vi "Airflow_Simulator_Main.vi"() -> ()   [LabVIEW 2025]
uses:
  controls/Tuners.ctl
  controls/Constants.ctl
  controls/Design_Results.ctl
  controls/UI Data.ctl
  Settings/Settings.ctl
  Acquisition/Hardware Configuration.ctl
  Acquisition/Signal Type.ctl
  Logging/Logging Configuration.ctl
  controls/UI State.ctl
  controls/State_Machine_Steps.ctl
  support/Message Queue/Enqueue Message (Single).vi
  support/Message Queue/Enqueue Message (Array).vi
  <vilib>/Utility/error.llb/Error Cluster From Error Code.vi
  <vilib>/ErrorRing/Error Ring.xnode
  Settings/Settings.lvlib
  support/Message Queue/Message Queue.lvlib
  Settings/Settings Dialog.vi
  support/User Event - Stop/User Event - Stop.lvlib
  Acquisition/Acquisition.lvlib
  Logging/Logging.lvlib
panel:
  in  "Tab Control":T1(tab)
  in  "Design Constants":T2={"P_amb (psia)"=14.7, "T_in (Deg F)"=530.0, "R_air (ft*lbf)/(lbm*R)"=53.35, "g_c (lbm*ft)/(lbf*s^2)"=32.17, "specific heat ratio"=1.4, "Viscousity (lbm)/(ft*s)"=1.21e-05, "Cd"=0.61, "Mass Flow (lbm/min) vs. Pressure Drop (inH2O) - Real Data"=[[0.5, 0.0149], [1.0, 0.0619], [1.5, 0.139], [2.0, 0.249], [2.5, 0.385], [3.5, 0.73]]} {"Mass Flow (lbm/min) vs. Pressure Drop (inH2O) - Real Data" format="%_3g"; "P_amb (psia)" format="%#_4g"}
  in  "Submit to DB":bool
  out "Design Results":T3 {"Design Results"."Optimized Inlet \nOrifice Diameter (in)" format="%#_3g"}
  in  "Tuners":T4 {"OAR" items=["0.92"=0.92, "0.93"=0.93, "0.94"=0.94, "0.95"=0.95, "0.96"=0.96]; "D_h (in)" items=["0.0625"=0.0625, "0.125"=0.125, "0.250"=0.25]; "Diameter (in)" min=0.1 max=6.0 scale=0.0..6.0 scale format="%#_3g"; "Length (in)" min=0.1 max=5.0 scale=0.0..6.0 scale format="%#_3g"; "Outlet Diameter (in)" min=0.1 max=5.0 scale=0.0..5.0 scale format="%#_3g"; "Inlet Diameter (in)" min=0.1 max=5.0 scale=0.0..5.0}
  in  "Start":bool
  in  "Settings":bool
  in  "Stop":bool
  in  "Exit":bool
  out "Status":string
  # "AIRFLOW SIMULATOR"
  # "Temperature_Tap"
  # "Pressure_Tap"
  # "Mass_flowrate"
  # "Outlet_Diameter"
  # "Inlet_Diameter"
  # "Pressure_Ambient"
  # "Pressure_Inlet"
  # "Pipe_Diameter"
  # "Temperature_Inlet"
  # "Honeycomb_Length"
  # "Temperature_Ambient"
  # "DESIGN PARAMETERS AND PROPERTIES"
  # "PIPE"
  # "ORIFICES"
  # "HONEYCOMB"
  # "AIR PROPERTIES"
  # "**Outlet_Diameter"
  # "**Pipe_Diameter"
  # "**D_h"
  # "Temperature_Inlet (Deg F) = 70"
  # "**Inlet_Diameter"
  # "**OAR"
  # "R_air (ft*lbf)/(lbm*R) = 53.35"
  # "Cd_orifice  = 0.61"
  # "**Honeycomb_Length"
  # "specific heat ratio = 1.40"
  # "Viscousity (lbm)/(ft*s) = 1.21E-5"
  # "**To Be Determine Using Design Mode"
  # "Pressure_Ambient (psia) = 14.7"
  # "Pressure_Inlet"
  # "Empirical Flow Path Data"
  # "Mass Flow\n (lbm/min)"
  # "Pressure Drop \n    (inH2O)"
  # "Simulator Fit"
  # "Empirical Fit"
  # "="
  # "P"
  # "* X"
  # "P"
  # "="
  # "* X"
  # "drop"
  # "drop"
  # "Honeycomb Parameters"
  # "Orifice Parameters"
  # "Pipe Parameters"
  # "AIRFLOW SIMULATOR"
  # "Mass_flowrate"
  # "Pipe_Diameter"
  # "Outlet_Diameter"
  # "Inlet_Diameter"
  # "Honeycomb_Length"
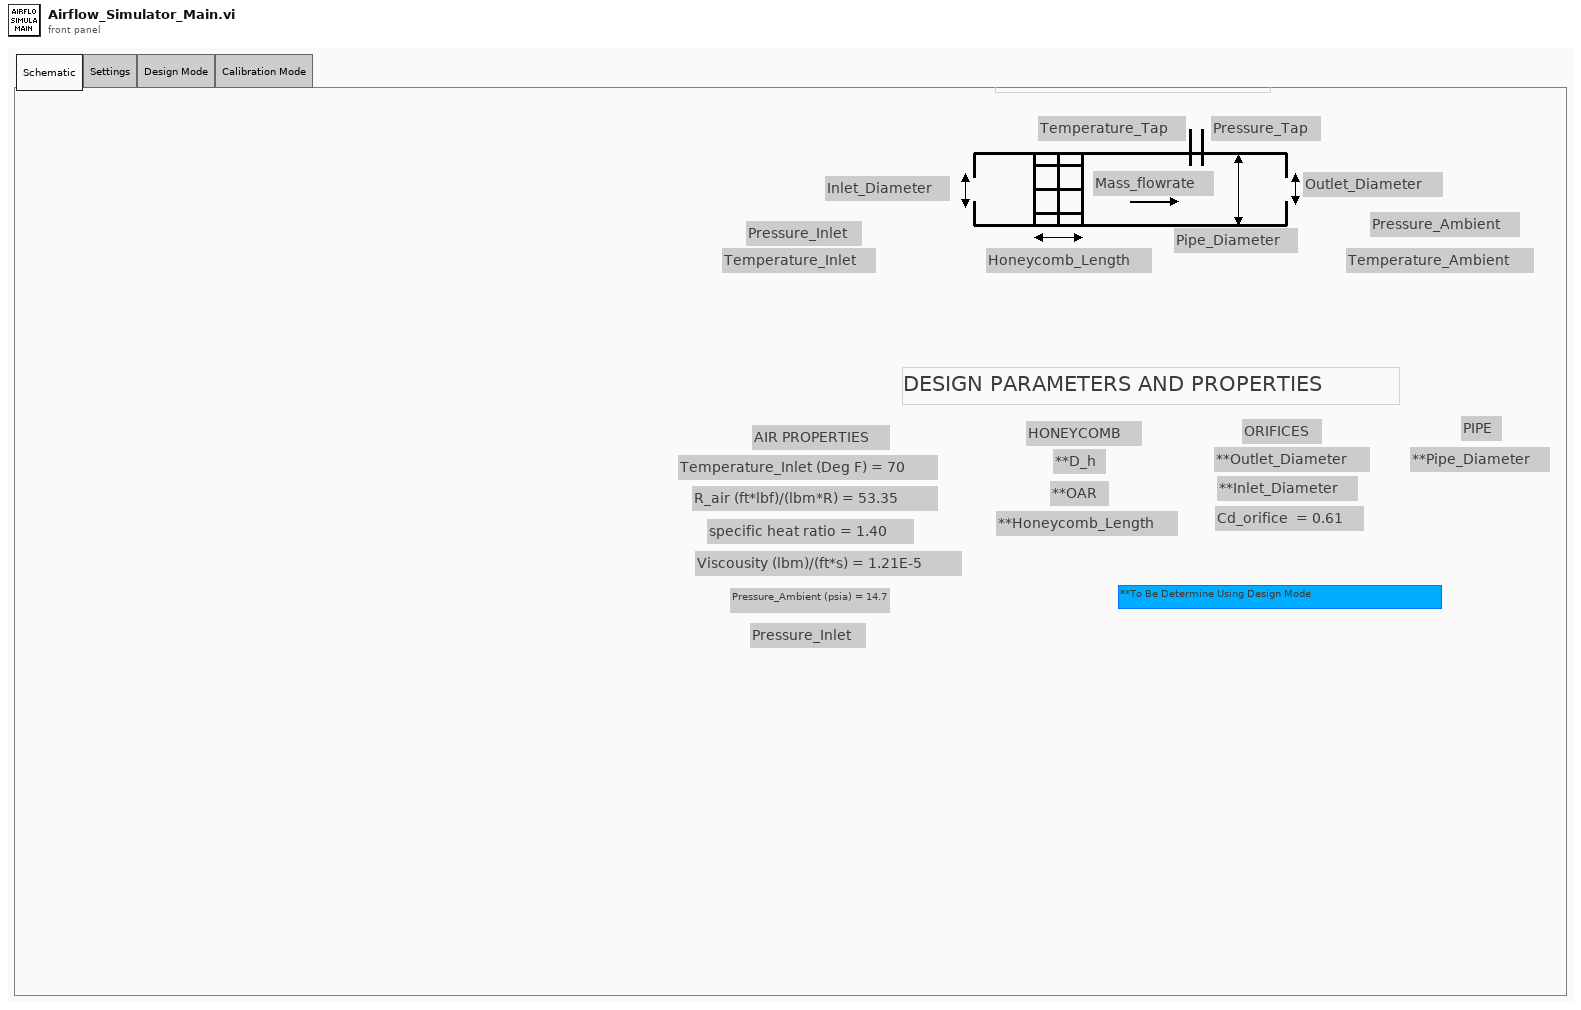
[diagram p1: front panel]
types:
  T1 = enum32{"Schematic", "Settings", "Design Mode", "Calibration Mode"}
  T2 = typedef "Constants.ctl" = cluster{"P_amb (psia)":dbl, "T_in (Deg F)":dbl, "R_air (ft*lbf)/(lbm*R)":dbl, "g_c (lbm*ft)/(lbf*s^2)":dbl, "specific heat ratio":dbl, "Viscousity (lbm)/(ft*s)":dbl, "Cd":dbl, "Mass Flow (lbm/min) vs. Pressure Drop (inH2O) - Real Data":dbl[][]}
  T3 = typedef "Design_Results.ctl" = cluster{"Design Results":cluster{"Model Validation: Simulated vs. Empirical Airflow Data":cluster{dbl[], dbl[]}[], "Amplitude - Empirical":string, "Power - Empirical":string, "Amplitude - Sim":string, "Power - Sim":string, "Flow Type":u32, "Optimized Inlet \nOrifice Diameter (in)":dbl, "Flow Type Name":string}}
  T4 = typedef "Tuners.ctl" = cluster{"Inlet Diameter (in)":dbl, "Outlet Diameter (in)":dbl, " Length (in)":dbl, "   Diameter (in)":dbl, "D_h (in)":dbl, "OAR":dbl, "Run Optimizer":bool}
  T5 = typedef "State_Machine_Steps.ctl" = enum16{"Init", "Event", "Design", "Calibrate", "Stop"}
  T6 = typedef "UI State.ctl" = enum16{"Idle", "Acquiring and Logging", "Waiting for Exit", "Waiting for Exit (Acq Stopped)", "Waiting for Exit (Log Stopped)", "Waiting for Stop", "Waiting for Stop (Acq Stopped)", "Waiting for Stop (Log Stopped)"}
  T7 = typedef "Settings.lvlib/Settings.ctl" = cluster{"Hardware Configuration":T8, "Logging Configuration":T10}
  T8 = typedef "Acquisition.lvlib/Hardware Configuration.ctl" = cluster{"HW Refnum <Replace Me>":string, "Signal Type <Replace Me>":T9}
  T9 = typedef "Acquisition.lvlib/Signal Type.ctl" = enum16{"Sine Wave", "Square with Noise"}
  T10 = typedef "Logging.lvlib/Logging Configuration.ctl" = cluster{"Log File Base Path":path, "TDMS File Reference":refnum<k34>}
  T11 = typedef "UI Data.ctl" = cluster{"Start Ref":refnum<vi>, "Stop Ref":refnum<vi>, "Settings Ref":refnum<vi>, "Exit Ref":refnum<vi>, "Status Ref":refnum<vi>, "Data Ref":refnum<vi>}
  T12 = typedef "Message Queue.lvlib/All Message Queues.ctl" = cluster{"UI":refnum<queue>, "Acquisition":refnum<queue>, "Logging":refnum<queue>, "Design":refnum<queue>, "Display":refnum<queue>, "Database":refnum<queue>}
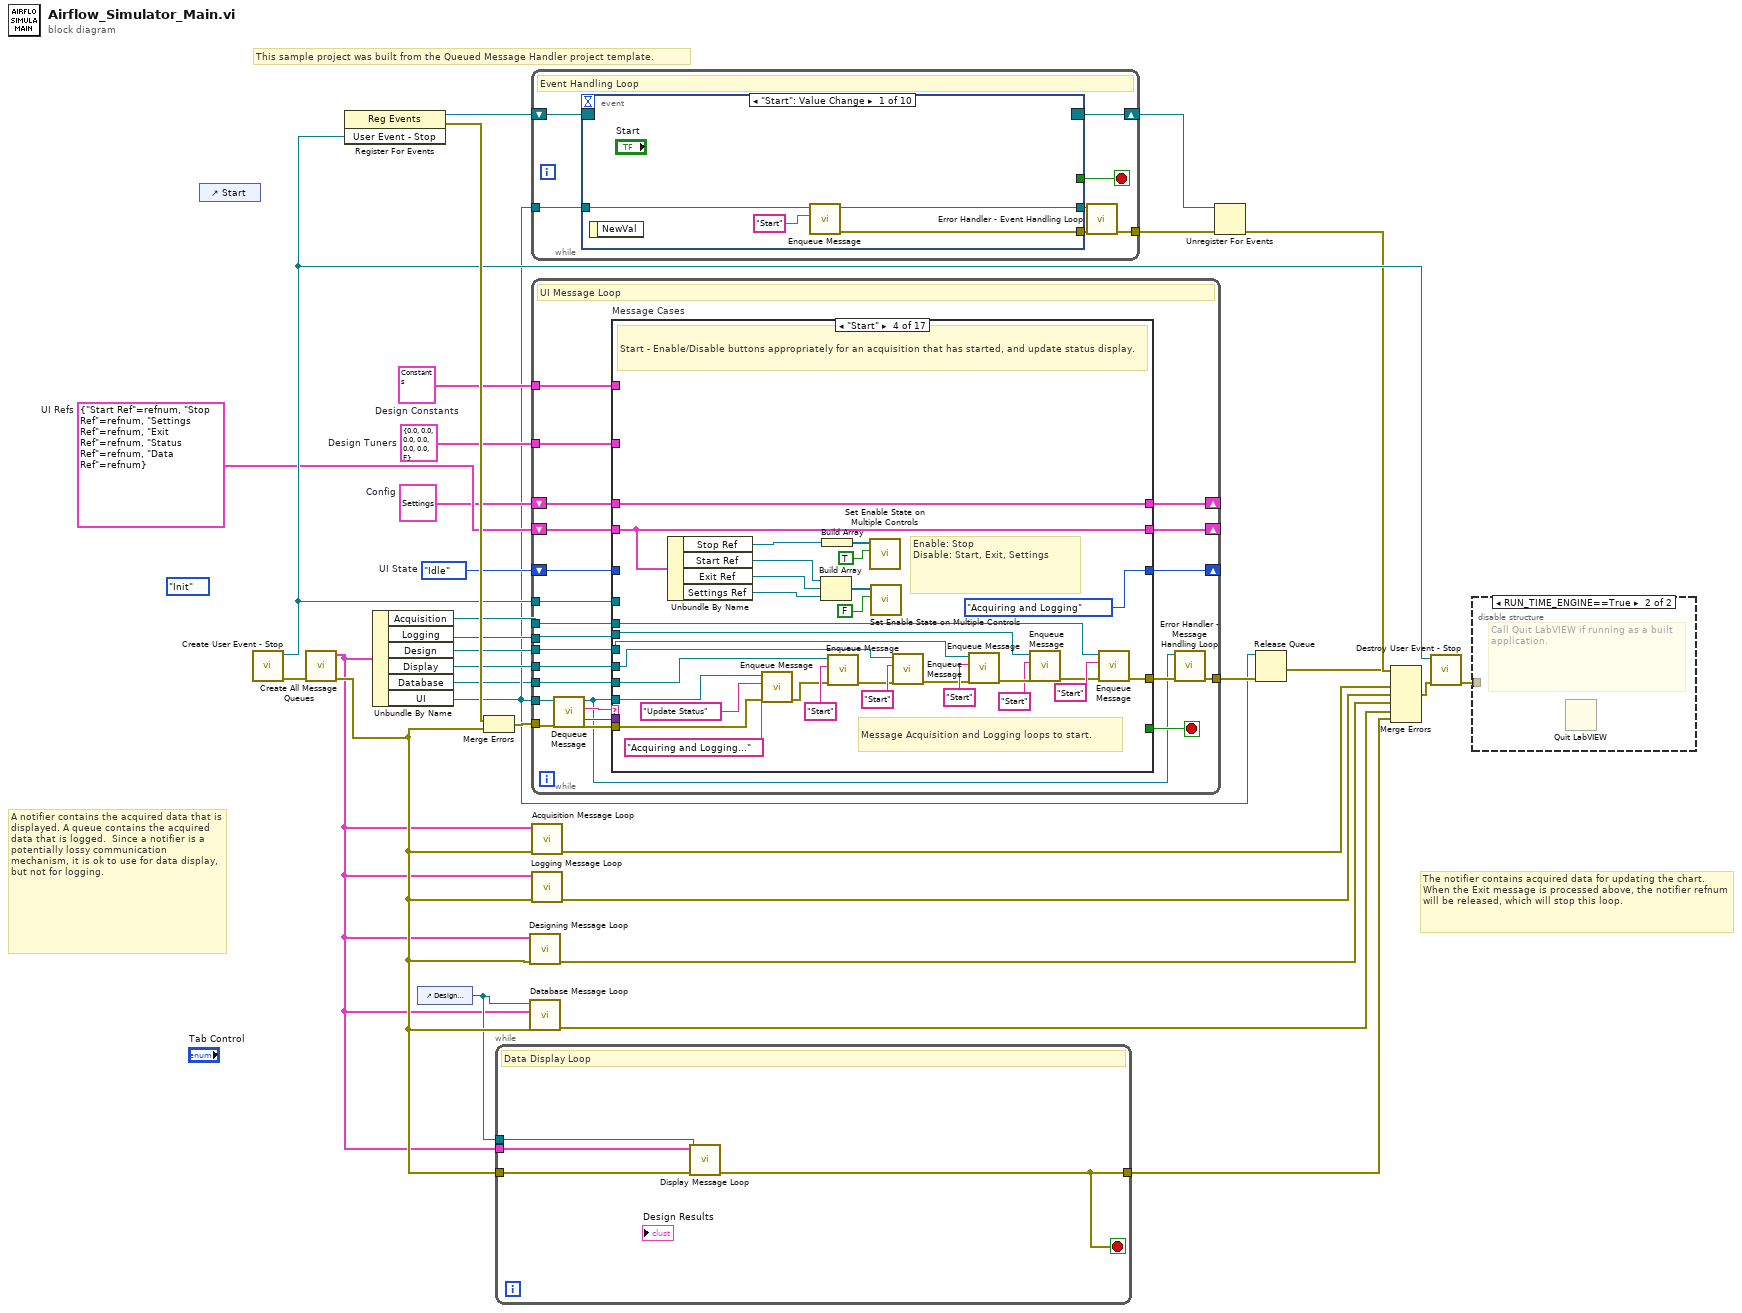
[diagram p0: block diagram]
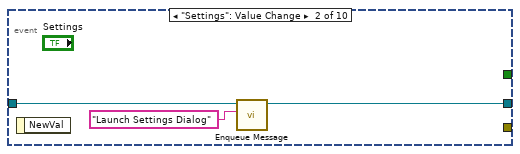
[diagram p3: hidden frame]
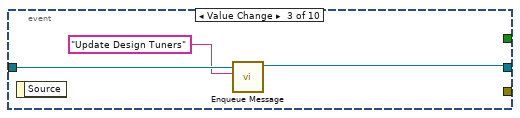
[diagram p4: hidden frame]
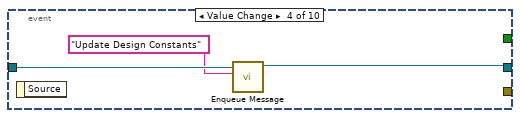
[diagram p5: hidden frame]
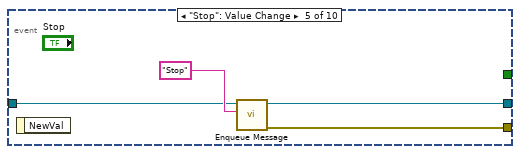
[diagram p6: hidden frame]
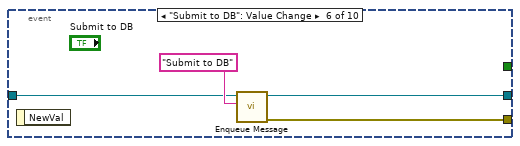
[diagram p7: hidden frame]
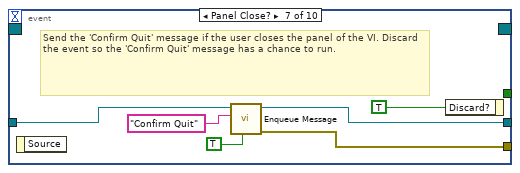
[diagram p8: hidden frame]
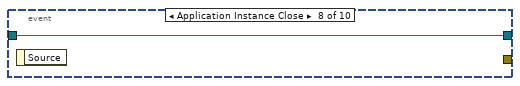
[diagram p9: hidden frame]
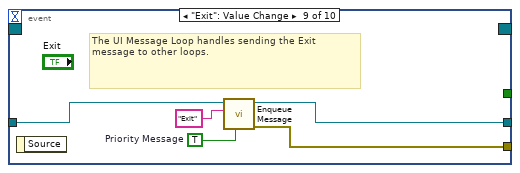
[diagram p10: hidden frame]
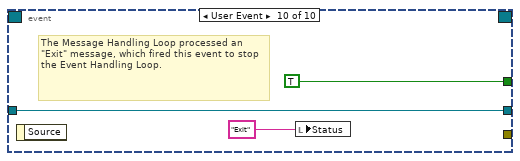
[diagram p11: hidden frame]
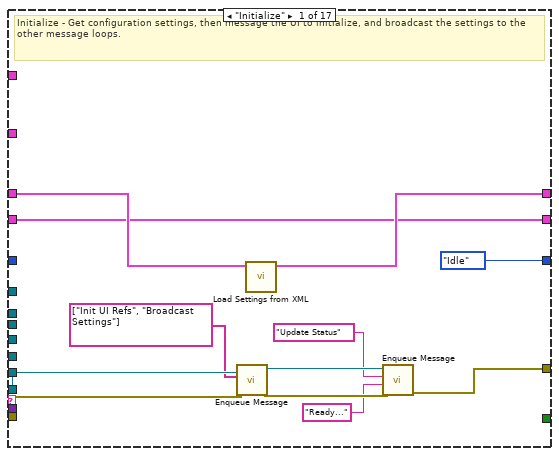
[diagram p12: hidden frame]
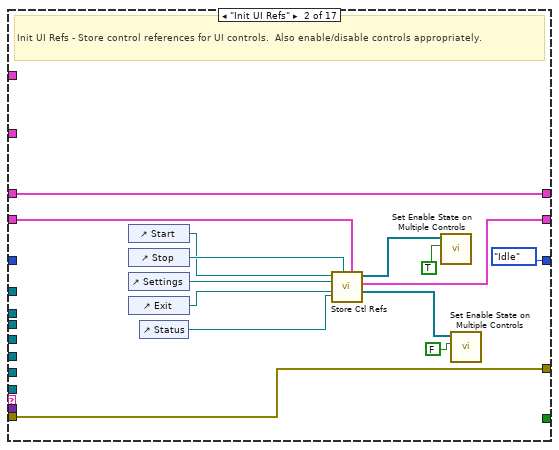
[diagram p13: hidden frame]
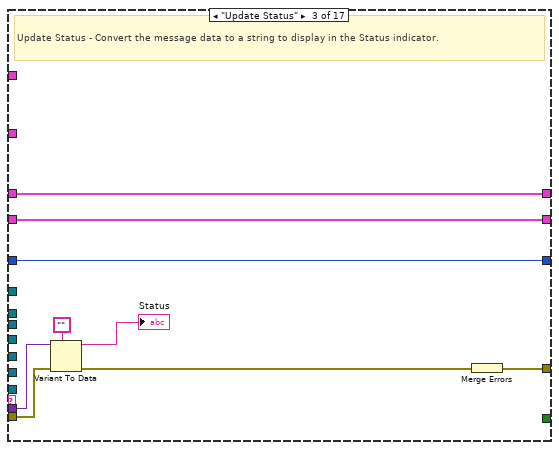
[diagram p14: hidden frame]
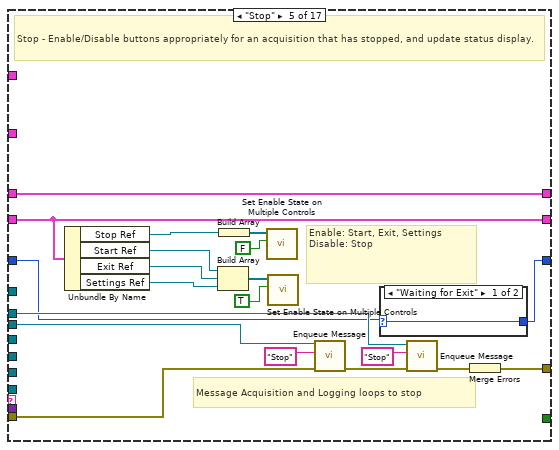
[diagram p15: hidden frame]
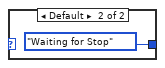
[diagram p16: hidden frame]
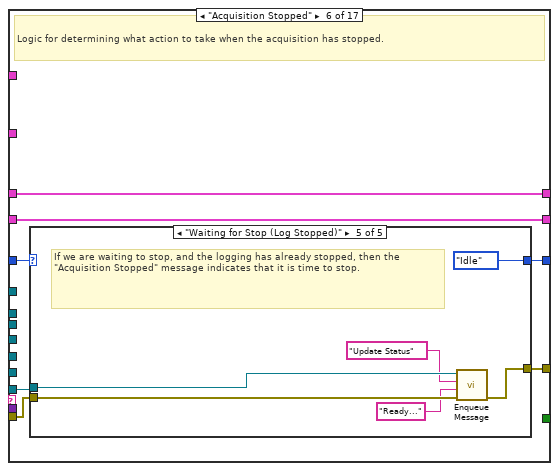
[diagram p17: hidden frame]
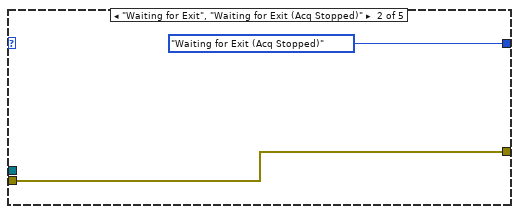
[diagram p19: hidden frame]
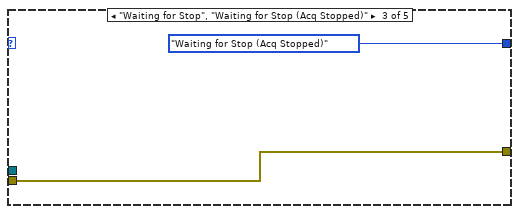
[diagram p20: hidden frame]
diagram:
  (unwired) State_Machine_Steps."Init" ("Enum")
  w12 = T2 {"P_amb (psia)"=14.7, "T_in (Deg F)"=70.0, "R_air (ft*lbf)/(lbm*R)"=53.35, "g_c (lbm*ft)/(lbf*s^2)"=32.17, "specific heat ratio"=1.4, "Viscousity (lbm)/(ft*s)"=1.21e-05, "Cd"=0.61, "Mass Flow (lbm/min) vs. Pressure Drop (inH2O) - Real Data"=[[0.5, 0.015], [1.0, 0.062], [1.5, 0.141], [2.0, 0.252], [2.5, 0.395], [3.5, 0.778]]}  # Design Constants
  w13 = T4 {"Inlet Diameter (in)"=0.0, "Outlet Diameter (in)"=0.0, " Length (in)"=0.0, "   Diameter (in)"=0.0, "D_h (in)"=0.0, "OAR"=0.0, "Run Optimizer"=FALSE}  # Design Tuners
  w25 = UI_State."Idle"  # UI State
  w19 = T7 {"Hardware Configuration"={"HW Refnum <Replace Me>"="", "Signal Type <Replace Me>"=enum."Sine Wave"}, "Logging Configuration"={"Log File Base Path"=path "", "TDMS File Reference"=refnum}}  # Config
  w22 = T11 {"Start Ref"=refnum, "Stop Ref"=refnum, "Settings Ref"=refnum, "Exit Ref"=refnum, "Status Ref"=refnum, "Data Ref"=refnum}  # UI Refs
  # "This sample project was built from the Queued Message Handler project template."
  # "A notifier contains the acquired data that is displayed. A queue contains the acquired data that is logged.  Since a notifier is a potentially lossy communication mechanism, it is ok to use for data display, but not for logging."
  # "The notifier contains acquired data for updating the chart. When the Exit message is processed above, the notifier refnum will be released, which will stop this loop."
  n1 = control-ref of="Start"() -> ()  [unwired: 1 out]
  n2 = call "Create User Event - Stop.vi"() -> ("error out"=w17:errorcluster, "User Event - Stop"=w29:refnum<user-event>)  [unwired: 10 in]
  n3 = call "Create All Message Queues.vi"("error in (no error)"=w17) -> ("error out"=w5:errorcluster, "Message Queues out"=w1:T12)  [unwired: 9 in]
  n4 = register-events(w29) -> (reference out=w28:refnum<event-registration>, error out=w31:errorcluster)  [unwired: 2 in]
  n5 = Unbundle By Name(w1) -> ("Acquisition"=w23:refnum<queue>, "Logging"=w24:refnum<queue>, "Design"=w11:refnum<queue>, "Display"=w9:refnum<queue>, "Database"=w6:refnum<queue>, "UI"=w7:refnum<queue>)
  n6 = control-ref of="Design Results"() -> (w2:refnum<vi>)
  n7 = Merge Errors(w31, w5) -> (w30:errorcluster)
  n8 = while "Data Display Loop" {
    tunnel: w1 -> [w35]
    tunnel: w5 -> [w34]
    tunnel: [w33] -> w4
    tunnel: w2 -> [w32]
    stop <- w33 stop-if-true
    # "Data Display Loop"
    n9 = call "Display Message Loop.vi"("error in (no error)"=w34, "Clust Refnum"=w32, "Message Queues"=w35) -> ("error out"=w33:errorcluster)  [unwired: 8 in]
  }
  n10 = call "Designing Message Loop.vi"("error in (no error)"=w5, "Message Queues"=w1) -> ("error out"=w10:errorcluster)  [unwired: 9 in]
  n11 = call "Database Message Loop.vi"("error in"=w5, "Message Queues"=w1, "Clust Refnum"=w2) -> ("error out"=w3:errorcluster)  [unwired: 8 in]
  n12 = while {
    tunnel: w7 -> [w41]
    tunnel: [w38] -> w15
    shift-right: [w40] -> w21
    shift-left: w28 -> [w42]
    stop <- w39 stop-if-true
    # "Event Handling Loop"
    n13 = event shown="[0] \"Start\": Value Change" {
      selector: w42 -> [_ _ _ _ _ _ _ _ _ _]
      dyn-events: [_ _ _ _ _ _ _ _ _ _] -> w40
      timeout: _ -> [_ _ _ _ _ _ _ _ _ _]
      tunnel: [_ _ _ _ _ _ _ _ _ TRUE ("Discard?")] -> w39
      tunnel: w41 -> [w46 w48 w52 w55 w58 w62 w67 w70 w72 w76]
      tunnel: [w44 _ _ _ w57 w61 w65 _ w75 _] -> w37
      tunnel: [w43 w47 w51 w54 w56 w60 w66 w70 w71 w76] -> w36
      event "Start": Value Change {
        n14 = event-data() -> ()  [unwired: 1 in, 1 out]
        n15 = call-poly "Enqueue Message.vi"("Message"="Start", "Message Queue"=w46) -> ("error out"=w44:errorcluster, "dup Message Queue"=w43:refnum<queue>)  [unwired: 8 in]
      }
      event "Settings": Value Change {
        n16 = event-data() -> ()  [unwired: 1 in, 1 out]
        n17 = call-poly "Enqueue Message.vi"("Message"="Launch Settings Dialog", "Message Queue"=w48) -> ("dup Message Queue"=w47:refnum<queue>)  [unwired: 8 in, 1 out]
      }
      event Value Change {
        n18 = event-data() -> ()  [unwired: 1 in, 1 out]
        n19 = call-poly "Enqueue Message.vi"("Message"="Update Design Tuners", "Message Queue"=w52) -> ("dup Message Queue"=w51:refnum<queue>)  [unwired: 8 in, 1 out]
      }
      event Value Change {
        n20 = event-data() -> ()  [unwired: 1 in, 1 out]
        n21 = call-poly "Enqueue Message.vi"("Message"="Update Design Constants", "Message Queue"=w55) -> ("dup Message Queue"=w54:refnum<queue>)  [unwired: 8 in, 1 out]
      }
      event "Stop": Value Change {
        n22 = event-data() -> ()  [unwired: 1 in, 1 out]
        n23 = call-poly "Enqueue Message.vi"("Message"="Stop", "Message Queue"=w58) -> ("error out"=w57:errorcluster, "dup Message Queue"=w56:refnum<queue>)  [unwired: 8 in]
      }
      event "Submit to DB": Value Change {
        n24 = event-data() -> ()  [unwired: 1 in, 1 out]
        n25 = call-poly "Enqueue Message.vi"("Message"="Submit to DB", "Message Queue"=w62) -> ("error out"=w61:errorcluster, "dup Message Queue"=w60:refnum<queue>)  [unwired: 8 in]
      }
      event Panel Close? {
        # "Send the 'Confirm Quit' message if the user closes the panel of the VI. Discard the event so the 'Confirm Quit' message has a chance to run."
        n26 = event-data() -> ()  [unwired: 1 in, 1 out]
        n27 = call-poly "Enqueue Message.vi"("Priority Message? (F)"=TRUE, "Message"="Confirm Quit", "Message Queue"=w67) -> ("error out"=w65:errorcluster, "dup Message Queue"=w66:refnum<queue>)  [unwired: 7 in]
        n28 = event-data("Discard?"=TRUE) -> ()  [unwired: 1 in, 1 out]
      }
      event Application Instance Close {
        n29 = event-data() -> ()  [unwired: 1 in, 1 out]
      }
      event "Exit": Value Change {
        w73 = TRUE  # Priority Message
        # "The UI Message Loop handles sending the Exit message to other loops."
        n30 = event-data() -> ()  [unwired: 1 in, 1 out]
        n31 = call-poly "Enqueue Message.vi"("Priority Message? (F)"=w73, "Message"="Exit", "Message Queue"=w72) -> ("error out"=w75:errorcluster, "dup Message Queue"=w71:refnum<queue>)  [unwired: 7 in]
      }
      event User Event {
        # "The Message Handling Loop processed an \"Exit\" message, which fired this event to stop the Event Handling Loop."
        n32 = event-data() -> ()  [unwired: 1 in, 1 out]
        n33 = local write "Status"("Exit" ("Exit String")) -> ()
      }
    }
    n34 = call "Error Handler - Event Handling Loop.vi"("error in (no error)"=w37, "Message Queue"=w36) -> ("dup error in"=w38:errorcluster)  [unwired: 8 in, 1 out]
  }
  n35 = while {
    tunnel: w29 -> [w100]
    shift-right: [w95] -> _
    shift-left: w19 -> [w94]
    shift-right: [w92] -> _
    shift-left: w22 -> [w93]
    tunnel: w23 -> [w91]
    tunnel: w24 -> [w90]
    shift-right: [w85] -> _
    shift-left: w25 -> [w86]
    tunnel: w30 -> [w99]
    tunnel: [w89] -> w14
    tunnel: w13 -> [w84]
    tunnel: w12 -> [w83]
    tunnel: w11 -> [w82]
    tunnel: w9 -> [w81]
    tunnel: w7 -> [w80]
    tunnel: w6 -> [w79]
    stop <- w101 stop-if-true
    # "UI Message Loop"
    n36 = call "Dequeue Message.vi"("error in (no error)"=w99, "Message Queue"=w80) -> ("error out"=w98:errorcluster, "Message Data"=w96:variant, "Message"=w97:string, "dup Message Queue"=w87:refnum<queue>)  [unwired: 6 in]
    n37 = case "Message Cases" shown="\"Start\"" w97 {
      selector: w97 -> [_ _ _ _ _ _ _ _ _ _ _ _ _ _ _ _ w351]
      tunnel: w87 -> [w105 _ _ w167 _ w192 w217 _ w252 _ w275 _ _ _ _ _ _]
      tunnel: w98 -> [w104 w127 w135 w166 w186 w193 w218 w246 w259 w266 w278 w306 w321 w331 w335 w344 _]
      tunnel: [w109 w127 w136 w144 w187 w190 w215 w251 w253 w269 w277 w316 w320 w330 w340 w349 w350] -> w88
      tunnel: [_ _ _ _ _ _ _ _ _ _ _ TRUE TRUE _ _ _ _] -> w101
      tunnel: w96 -> [_ _ w134 _ _ _ _ _ _ w270 _ w304 _ _ _ _ _]
      tunnel: w100 -> [_ _ _ _ _ _ _ _ _ _ _ w317 _ _ _ _ _]
      tunnel: [w112 w126 w130 w165 w185 w196 w221 w249 w257 w274 w281 w315 w325 w329 w339 w348 w354] -> w95
      tunnel: w94 -> [w113 w126 w130 w165 w185 w196 w221 w249 w260 w274 w281 w315 w325 w329 w339 w348 w354]
      tunnel: w93 -> [w106 w114 w129 w162 w184 w195 w220 w245 w255 w273 w280 w314 w324 w328 w338 w347 w353]
      tunnel: [w106 w124 w129 w162 w184 w195 w220 w245 w255 w273 w280 w314 w324 w328 w338 w347 w353] -> w92
      tunnel: w91 -> [_ _ _ w145 w171 _ _ w244 _ _ _ w313 _ _ _ _ _]
      tunnel: w90 -> [_ _ _ w143 w174 _ _ w243 _ _ _ w312 _ _ _ _ _]
      tunnel: w86 -> [_ _ w128 _ w168 w194 w219 w242 w254 w268 w279 _ _ w327 w337 w346 w352]
      tunnel: [UI_State."Idle" ("UI State") UI_State."Idle" ("UI State") w128 UI_State."Acquiring and Logging" ("UI State") w169 w191 w216 w242 w254 w268 w276 UI_State."Idle" ("UI State") UI_State."Idle" ("UI State") w327 w337 w346 w352] -> w85
      tunnel: w84 -> [_ _ _ _ _ _ _ _ _ _ _ _ _ _ _ _ _]
      tunnel: w83 -> [_ _ _ _ _ _ _ _ _ _ _ _ _ _ _ _ _]
      tunnel: w82 -> [_ _ _ w142 _ _ _ _ _ _ _ _ _ _ w336 w343 _]
      tunnel: w81 -> [_ _ _ w141 _ _ _ _ _ _ _ _ _ _ _ _ _]
      tunnel: w79 -> [_ _ _ w137 _ _ _ _ _ _ _ _ w319 _ _ _ _]
      frame "Initialize" {
        # "Initialize - Get configuration settings, then message the UI to initialize, and broadcast the settings to the other message loops."
        n38 = call-poly "Enqueue Message.vi"("error in (no error)"=w104, "Message Array"=string[] ["Init UI Refs", "Broadcast Settings"], "Message Queue"=w105) -> ("error out"=w111:errorcluster, "dup Message Queue"=w110:refnum<queue>)  [unwired: 7 in]
        n39 = call "Load Settings from XML.vi"("Settings in"=w113) -> ("Settings out"=w112:T7)  [unwired: 9 in, 1 out]
        n40 = call-poly "Enqueue Message.vi"("error in (no error)"=w111, "Message Data"="Ready..." ("Ready..."), "Message"="Update Status", "Message Queue"=w110) -> ("error out"=w109:errorcluster)  [unwired: 6 in, 1 out]
      }
      frame "Init UI Refs" {
        # "Init UI Refs - Store control references for UI controls.  Also enable/disable controls appropriately."
        n41 = control-ref of="Start"() -> (w118:refnum<vi>)
        n42 = control-ref of="Stop"() -> (w119:refnum<vi>)
        n43 = control-ref of="Settings"() -> (w117:refnum<vi>)
        n44 = control-ref of="Exit"() -> (w116:refnum<vi>)
        n45 = control-ref of="Status"() -> (w125:refnum<vi>)
        n46 = call "Store Ctl Refs.vi"("UI Refs in"=w114, "Status"=w125, "Stop"=w119, "Exit"=w116, "Settings"=w117, "Start"=w118) -> ("Disable"=w121:refnum<vi>[], "UI Refs out"=w124:T11, "Enable"=w122:refnum<vi>[])  [unwired: 3 in]
        n47 = call "Set Enable State on Multiple Controls.vi"("Enable?"=TRUE, "Controls"=w122) -> ()  [unwired: 10 in]
        n48 = call "Set Enable State on Multiple Controls.vi"("Enable?"=FALSE, "Controls"=w121) -> ()  [unwired: 10 in]
      }
      frame "Update Status" {
        # "Update Status - Convert the message data to a string to display in the Status indicator."
        n49 = Variant To Data(error in=w135, type="", Variant=w134) -> (data=→"Status":string, error out=w132:errorcluster)
        n50 = Merge Errors(w132) -> (w136:errorcluster)
      }
      frame "Start" {
        # "Message Acquisition and Logging loops to start."
        # "Enable: Stop\nDisable: Start, Exit, Settings"
        # "Start - Enable/Disable buttons appropriately for an acquisition that has started, and update status display."
        n51 = Unbundle By Name(w162) -> ("Stop Ref"=w157:refnum<vi>, "Start Ref"=w156:refnum<vi>, "Exit Ref"=w155:refnum<vi>, "Settings Ref"=w154:refnum<vi>)
        n52 = call-poly "Enqueue Message.vi"("error in (no error)"=w166, "Message Data"="Acquiring and Logging..." ("Acquiring and Logging..."), "Message"="Update Status", "Message Queue"=w167) -> ("error out"=w139:errorcluster)  [unwired: 6 in, 1 out]
        n53 = Build Array(w156, w155, w154) -> (w160:refnum<vi>[])
        n54 = Build Array(w157) -> (w159:refnum<vi>[])
        n55 = call-poly "Enqueue Message.vi"("error in (no error)"=w139, "Message"="Start", "Message Queue"=w137) -> ("error out"=w138:errorcluster)  [unwired: 7 in, 1 out]
        n56 = call "Set Enable State on Multiple Controls.vi"("Enable?"=TRUE, "Controls"=w159) -> ()  [unwired: 10 in]
        n57 = call "Set Enable State on Multiple Controls.vi"("Enable?"=FALSE, "Controls"=w160) -> ()  [unwired: 10 in]
        n58 = call-poly "Enqueue Message.vi"("error in (no error)"=w138, "Message"="Start", "Message Queue"=w141) -> ("error out"=w146:errorcluster)  [unwired: 7 in, 1 out]
        n59 = call-poly "Enqueue Message.vi"("error in (no error)"=w146, "Message"="Start", "Message Queue"=w142) -> ("error out"=w152:errorcluster)  [unwired: 7 in, 1 out]
        n60 = call-poly "Enqueue Message.vi"("error in (no error)"=w152, "Message"="Start", "Message Queue"=w143) -> ("error out"=w148:errorcluster)  [unwired: 7 in, 1 out]
        n61 = call-poly "Enqueue Message.vi"("error in (no error)"=w148, "Message"="Start", "Message Queue"=w145) -> ("error out"=w144:errorcluster)  [unwired: 7 in, 1 out]
      }
      frame "Stop" {
        # "Message Acquisition and Logging loops to stop"
        # "Enable: Start, Exit, Settings\nDisable: Stop"
        # "Stop - Enable/Disable buttons appropriately for an acquisition that has stopped, and update status display."
        n62 = Unbundle By Name(w184) -> ("Stop Ref"=w179:refnum<vi>, "Start Ref"=w178:refnum<vi>, "Exit Ref"=w177:refnum<vi>, "Settings Ref"=w176:refnum<vi>)
        n63 = Build Array(w178, w177, w176) -> (w182:refnum<vi>[])
        n64 = Build Array(w179) -> (w181:refnum<vi>[])
        n65 = call "Set Enable State on Multiple Controls.vi"("Enable?"=FALSE, "Controls"=w181) -> ()  [unwired: 10 in]
        n66 = call "Set Enable State on Multiple Controls.vi"("Enable?"=TRUE, "Controls"=w182) -> ()  [unwired: 10 in]
        n67 = call-poly "Enqueue Message.vi"("error in (no error)"=w186, "Message"="Stop", "Message Queue"=w174) -> ("error out"=w173:errorcluster)  [unwired: 7 in, 1 out]
        n68 = case shown="\"Waiting for Exit\"" w168 {
          selector: w168 -> [w188 _]
          tunnel: [w188 UI_State."Waiting for Stop" ("UI State")] -> w169
          frame "Waiting for Exit" {
          }
          frame Default {
          }
        }
        n69 = call-poly "Enqueue Message.vi"("error in (no error)"=w173, "Message"="Stop", "Message Queue"=w171) -> ("error out"=w172:errorcluster)  [unwired: 7 in, 1 out]
        n70 = Merge Errors(w172) -> (w187:errorcluster)
      }
      frame "Acquisition Stopped" {
        # "Logic for determining what action to take when the acquisition has stopped."
        n71 = case shown="\"Waiting for Stop (Log Stopped)\"" w194 {
          selector: w194 -> [w198 _ _ _ _]
          tunnel: w193 -> [w197 w200 w202 w208 w214]
          tunnel: w192 -> [_ _ _ w203 w211]
          tunnel: [w198 UI_State."Waiting for Exit (Acq Stopped)" ("UI State") UI_State."Waiting for Stop (Acq Stopped)" ("UI State") UI_State."Idle" ("UI State") UI_State."Idle" ("UI State")] -> w191
          tunnel: [w197 w200 w202 w207 w212] -> w190
          frame Default {
          }
          frame "Waiting for Exit", "Waiting for Exit (Acq Stopped)" {
          }
          frame "Waiting for Stop", "Waiting for Stop (Acq Stopped)" {
          }
          frame "Waiting for Exit (Log Stopped)" {
            # "If we are waiting to exit, and the logging has already stopped, then the \"Acquisition Stopped\" message indicates that it is time to exit."
            n72 = call-poly "Enqueue Message.vi"("Priority Message? (F)"=TRUE, "error in (no error)"=w208, "Message"="Exit", "Message Queue"=w203) -> ("error out"=w207:errorcluster)  [unwired: 6 in, 1 out]
          }
          frame "Waiting for Stop (Log Stopped)" {
            # "If we are waiting to stop, and the logging has already stopped, then the \"Acquisition Stopped\" message indicates that it is time to stop."
            n73 = call-poly "Enqueue Message.vi"("error in (no error)"=w214, "Message Data"="Ready..." ("Ready..."), "Message"="Update Status", "Message Queue"=w211) -> ("error out"=w212:errorcluster)  [unwired: 6 in, 1 out]
          }
        }
      }
      frame "Logging Stopped" {
        # "Logic for determining what action to take when the logging has stopped."
        n74 = case shown="\"Waiting for Exit\", \"Waiting for Exit (Log Stopped)\"" w219 {
          selector: w219 -> [w223 _ _ _ _]
          tunnel: w218 -> [w222 w225 w227 w233 w236]
          tunnel: w217 -> [_ _ _ w231 w235]
          tunnel: [w223 UI_State."Waiting for Exit (Log Stopped)" ("UI State") UI_State."Waiting for Stop (Log Stopped)" ("UI State") UI_State."Idle" ("UI State") UI_State."Idle" ("UI State")] -> w216
          tunnel: [w222 w225 w227 w232 w234] -> w215
          frame Default {
          }
          frame "Waiting for Exit", "Waiting for Exit (Log Stopped)" {
          }
          frame "Waiting for Stop", "Waiting for Stop (Log Stopped)" {
          }
          frame "Waiting for Exit (Acq Stopped)" {
            # "If we are waiting to exit, and the acquisition has already stopped, then the \"Logging Stopped\" message indicates that it is time to exit."
            n75 = call-poly "Enqueue Message.vi"("Priority Message? (F)"=TRUE, "error in (no error)"=w233, "Message"="Exit", "Message Queue"=w231) -> ("error out"=w232:errorcluster)  [unwired: 6 in, 1 out]
          }
          frame "Waiting for Stop (Acq Stopped)" {
            # "If we are waiting to stop, and the acquisition has already stopped, then the \"Logging Stopped\" message indicates that it is time to stop."
            n76 = call-poly "Enqueue Message.vi"("error in (no error)"=w236, "Message Data"="Ready..." ("Ready..."), "Message"="Update Status", "Message Queue"=w235) -> ("error out"=w234:errorcluster)  [unwired: 6 in, 1 out]
          }
        }
      }
      frame "Broadcast settings" {
        w241 = "Update Settings" ("Message")
        # "Broadcast settings - Send the 'Update Settings' message to the Logging and Acquisition message loops."
        n77 = Unbundle By Name(w249) -> ("Hardware Configuration"=w248:T8, "Logging Configuration"=w247:T10)
        n78 = call-poly "Enqueue Message.vi"("Message Data"=w248, "Message"=w241, "Message Queue"=w244) -> ("error out"=w250:errorcluster)  [unwired: 7 in, 1 out]
        n79 = call-poly "Enqueue Message.vi"("error in (no error)"=w250, "Message Data"=w247, "Message"=w241, "Message Queue"=w243) -> ("error out"=w240:errorcluster)  [unwired: 6 in, 1 out]
        n80 = Merge Errors(w240, w246) -> (w251:errorcluster)
      }
      frame "Launch Settings Dialog" {
        # "Launch Settings Dialog - Launch the Settings Dialog when the user clicks the 'Settings' button."
        n81 = call-by-ref "?"("error in (no error)"=w259, "Settings in"=w260) -> ("error out"=w256:errorcluster, "Cancelled?"=w258:bool, "Settings out"=w257:T7)  [unwired: 8 in, 3 out]
        n82 = case shown="False" w258 {
          tunnel: w252 -> [w264 _]
          tunnel: w256 -> [w263 w265]
          tunnel: [w262 w265] -> w253
          frame False {
            n83 = call-poly "Enqueue Message.vi"("error in (no error)"=w263, "Message"="Broadcast Settings", "Message Queue"=w264) -> ("error out"=w262:errorcluster)  [unwired: 7 in, 1 out]
          }
          frame True {
          }
        }
      }
      frame "Error" {
        # "Error - Display an error dialog. This message is sent by the \"Error Handler\" VIs at the end of other loops in this application."
        n84 = Variant To Data(error in=w266, type=errorcluster {"status"=FALSE, "code"=0, "source"=""} ("error constant"), Variant=w270) -> (data=w267:errorcluster, error out=w271:errorcluster)
        n85 = call <vilib>:"Simple Error Handler.vi"("error in (no error)"=w267) -> ()  [unwired: 4 in, 5 out]
        n86 = Merge Errors(w271) -> (w269:errorcluster)
      }
      frame "Confirm Quit" {
        # "Confirm Quit - Message that can confirm whether or not the user wants to exit the application."
        n87 = case shown="\"Acquiring and Logging\"" w279 {
          tunnel: w275 -> [w287 w291]
          tunnel: w278 -> [w286 w290]
          tunnel: [w285 w289] -> w277
          tunnel: [UI_State."Idle" ("UI State") w288] -> w276
          frame Default {
            # "If 'Confirm Quit' comes in while the system is idle, there is no need for a confirmation message."
            n88 = call-poly "Enqueue Message.vi"("Priority Message? (F)"=TRUE, "error in (no error)"=w286, "Message"="Exit", "Message Queue"=w287) -> ("error out"=w285:errorcluster)  [unwired: 6 in, 1 out]
          }
          frame "Acquiring and Logging" {
            n89 = Two Button Dialog(message="Are you sure you want to quit while the acquisition is running?" ("Confirm Quit Message"), 1:"No" ("No"), 2:"Yes" ("Yes")) -> (T button?=w292:bool)
            n90 = case shown="True" w292 {
              tunnel: w291 -> [_ w301]
              tunnel: w290 -> [w297 w302]
              tunnel: [w297 w300] -> w289
              tunnel: [UI_State."Acquiring and Logging" ("UI State") UI_State."Waiting for Exit" ("UI State")] -> w288
              frame False {
                # "User did not want to quit."
              }
              frame True {
                n91 = call-poly "Enqueue Message.vi"("error in (no error)"=w302, "Message"="Stop", "Message Queue"=w301) -> ("error out"=w300:errorcluster)  [unwired: 7 in, 1 out]
              }
            }
          }
        }
      }
      frame "Exit" {
        w308 = TRUE ("Priority Message? (F)")
        w309 = "Exit" ("Message")
        # "Popup an error dialog if 'Exit' was called as a result of an error."
        # "Stop the VI"
        # "Exit - Send Exit messages to the Acquisition and Logging loops, and fire the user event to stop the Event Handling Loop."
        n92 = Variant To Data(type=errorcluster {"status"=FALSE, "code"=0, "source"=""} ("error constant"), Variant=w304) -> (data=w303:errorcluster)  [unwired: 1 in, 1 out]
        n93 = call <vilib>:"Simple Error Handler.vi"("error in (no error)"=w303) -> ()  [unwired: 4 in, 5 out]
        n94 = call-poly "Enqueue Message.vi"("Priority Message? (F)"=w308, "error in (no error)"=w306, "Message"=w309, "Message Queue"=w313) -> ("error out"=w310:errorcluster)  [unwired: 6 in, 1 out]
        n95 = call-poly "Enqueue Message.vi"("Priority Message? (F)"=w308, "error in (no error)"=w310, "Message"=w309, "Message Queue"=w312) -> ("error out"=w307:errorcluster)  [unwired: 6 in, 1 out]
        n96 = call "Fire User Event - Stop.vi"("error in (no error)"=w307, "User Event - Stop"=w317) -> ("error out"=w316:errorcluster)  [unwired: 9 in]
      }
      frame "Submit to DB" {
        # "Stop the VI"
        # "Exit - Send Exit messages to the Acquisition and Logging loops, and fire the user event to stop the Event Handling Loop."
        n97 = call-poly "Enqueue Message.vi"("error in (no error)"=w321, "Message"="Submit to DB", "Message Queue"=w319) -> ("error out"=w320:errorcluster)  [unwired: 7 in, 1 out]
      }
      frame "---Copy This Frame---" {
        # "Duplicate this frame when creating new messages.  Change this comment in the duplicated frame to describe this message."
        n98 = Merge Errors(w331) -> (w330:errorcluster)
      }
      frame "Update Design Tuners" {
        # "Duplicate this frame when creating new messages.  Change this comment in the duplicated frame to describe this message."
        n99 = call-poly "Enqueue Message.vi"("error in (no error)"=w335, "Message Data"="Tuners", "Message"="Update Design Tuners", "Message Queue"=w336) -> ("error out"=w333:errorcluster)  [unwired: 6 in, 1 out]
        n100 = Merge Errors(w333) -> (w340:errorcluster)
      }
      frame "Update Design Constants" {
        # "Duplicate this frame when creating new messages.  Change this comment in the duplicated frame to describe this message."
        n101 = call-poly "Enqueue Message.vi"("error in (no error)"=w344, "Message Data"="Design Constants", "Message"="Update Design Constants", "Message Queue"=w343) -> ("error out"=w345:errorcluster)  [unwired: 6 in, 1 out]
        n102 = Merge Errors(w345) -> (w349:errorcluster)
      }
      frame Default {
        # "'Default' case only runs if there is a message that isn't defined in any of the other cases.  Output a programming error."
        n103 = xnode "Error Ring"("parameter 0"=w351) -> ("error out"=w350:errorcluster)
      }
    }
    n104 = call "Error Handler - Message Handling Loop.vi"("error in (no error)"=w88, "Message Queue"=w87) -> ("dup error in"=w89:errorcluster)  [unwired: 8 in, 1 out]
  }
  n105 = call "Acquisition Message Loop.vi"("error in (no error)"=w5, "Message Queues"=w1) -> ("error out"=w16:errorcluster)  [unwired: 9 in]
  n106 = call "Logging Message Loop.vi"("error in (no error)"=w5, "Message Queues"=w1) -> ("error out"=w18:errorcluster)  [unwired: 9 in]
  n107 = Unregister For Events(event registration refnum=w21, error in=w15) -> (error out=w20:errorcluster)
  n108 = Release Queue(queue=w7, error in (no error)=w14) -> (error out=w8:errorcluster)  [unwired: 1 in, 2 out]
  n109 = Merge Errors(w20, w8, w16, w18, w10, w3, w4) -> (w26:errorcluster)
  n110 = call "Destroy User Event - Stop.vi"("error in (no error)"=w26, "User Event - Stop"=w29) -> ("error out"=w27:errorcluster)  [unwired: 9 in]
  n111 = disable-structure shown="RUN_TIME_ENGINE==True" {
    disable-tunnel: w27 -> [_ _]
    frame condition #0 (active) {
    }
    frame condition #1 {
      # "Call Quit LabVIEW if running as a built application."
      n112 = Quit LabVIEW() -> ()  [unwired: 1 in]
    }
  }
